vi "Binary number generator.vi"() -> ()   [LabVIEW 2009]
panel:
  out "16bit integer":i16[](array[numeric])
  in  "Bits":i32
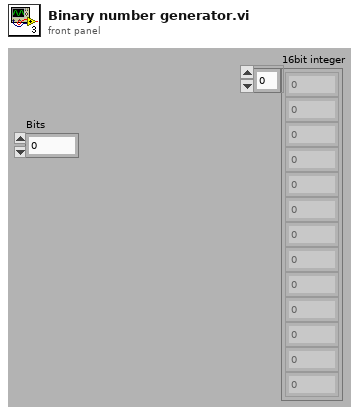
[diagram p1: front panel]
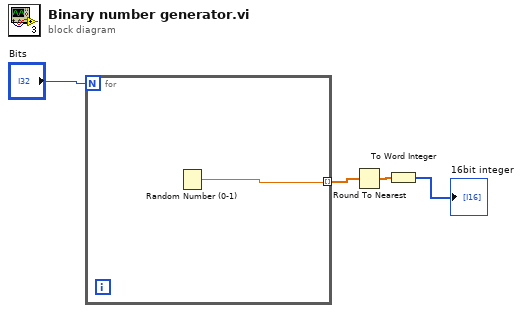
[diagram p0: block diagram]
diagram:
  n1 = for {
    N: "Bits" -> [_]
    tunnel: [w5] -> w3 mode=indexing
    n2 = Random Number (0-1)() -> (number: 0 to 1=w5:dbl)
  }
  n3 = Round To Nearest(number=w3) -> (nearest integer value=w2:dbl[])
  n4 = To Word Integer(number=w2) -> (16bit integer=→"16bit integer":i16[])
